vi "XY Graph Default X Step.vi"(6 "Get (F)/Set":bool, 8 "Error In":errorcluster, 11 "Default X Step":dbl) -> (0 "Error Out":errorcluster, 3 "Default X Step":dbl)   [LabVIEW 2021, in "XY Graph Add-Ons.lvlib"]
uses:
  XY Graph Add-Ons.lvlib
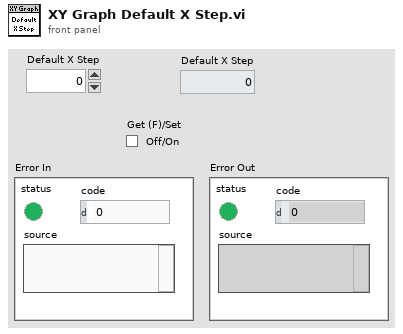
[diagram p1: front panel]
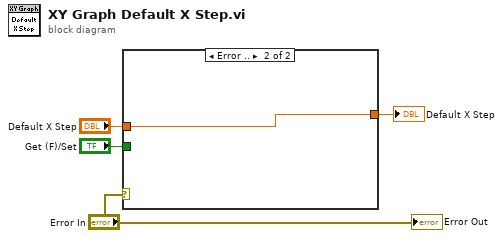
[diagram p0: block diagram]
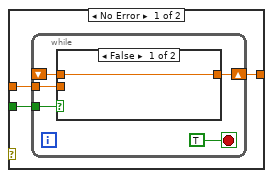
[diagram p2: hidden frame]
diagram:
  n1 = case shown="Error .." "Error In" {
    tunnel: "Get (F)/Set" -> [w7 _]
    tunnel: "Default X Step" -> [w6 w15]
    tunnel: [w5 w15] -> w2
    frame No Error {
      n2 = while {
        tunnel: w7 -> [w11]
        shift-right: [w10] -> w5
        shift-left: _ -> [w8]
        tunnel: w6 -> [w9]
        stop <- TRUE stop-if-true
        n3 = case shown="False" w11 {
          tunnel: [w13 w14] -> w10
          tunnel: w9 -> [_ w14]
          tunnel: w8 -> [w13 _]
          frame False {
          }
          frame True {
          }
        }
      }
    }
    frame Error {
    }
  }
  "Default X Step" <- w2
  "Error Out" <- "Error In"
